vi "Scale Change for Output.vi"(7 "WFChart Refnum":refnum<vi>, 8 "Min Out":dbl, 9 "Max Out":dbl, 10 "Boolean":bool, 11 "Output Unit":enum16{"%", "EGU"}(ring)) -> ()   [LabVIEW 2023]
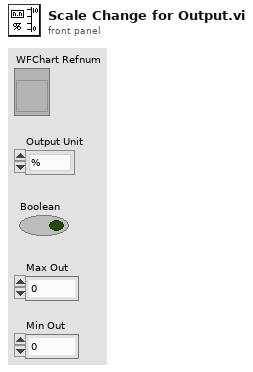
[diagram p1: front panel]
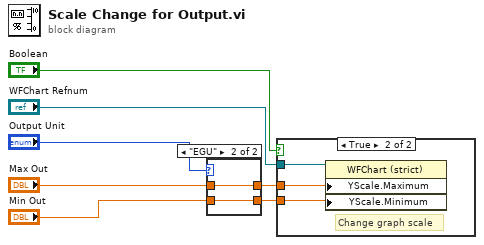
[diagram p0: block diagram]
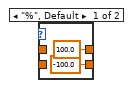
[diagram p3: hidden frame]
diagram:
  n1 = case shown="\"EGU\"" "Output Unit" {
    tunnel: [100.0 ("Data Range:Maximum") w11] -> w3
    tunnel: [-100.0 ("Data Range:Minimum") w10] -> w4
    tunnel: "Max Out" -> [_ w11]
    tunnel: "Min Out" -> [_ w10]
    frame "%", Default {
    }
    frame "EGU" {
    }
  }
  n2 = case shown="True" "Boolean" {
    tunnel: w3 -> [_ w14]
    tunnel: w4 -> [_ w13]
    tunnel: "WFChart Refnum" -> [_ w12]
    frame False {
    }
    frame True {
      # "Change graph scale"
      n3 = property on="Property Node" class="WFChart (strict)"(reference=w12, "YScale.Maximum"=w14, "YScale.Minimum"=w13) -> ()  [unwired: 1 in, 2 out]
    }
  }
